vi "Set LEDs.vi"(8 "error in (no error)":errorcluster, 10 "LED Array":u32[][](array[colorbox]), 11 "LINX-SenseHat in":refnum<class "LINX-SenseHat.lvclass">) -> (0 "error out":errorcluster, 3 "LINX-SenseHat out":refnum<class "LINX-SenseHat.lvclass">)   [LabVIEW 2020, in "LINX-SenseHat.lvclass"]
uses:
  LINX-SenseHat.lvclass
  LINX-SenseHat.lvclass/LINX-SenseHat.ctl
  LINX I2C/LINX I2C.lvclass
panel:
  out "size(s)":i32
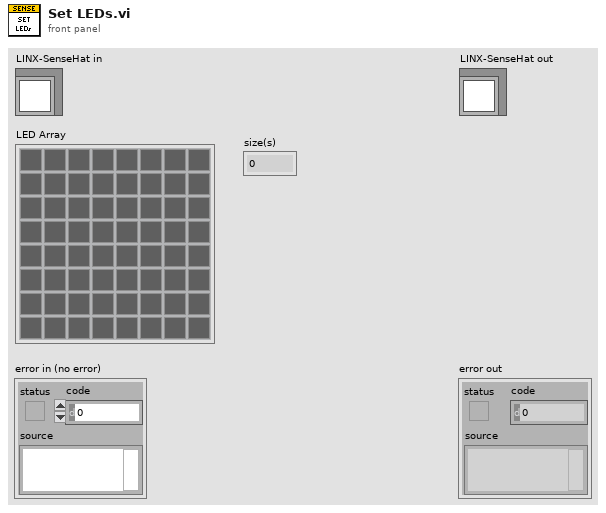
[diagram p1: front panel]
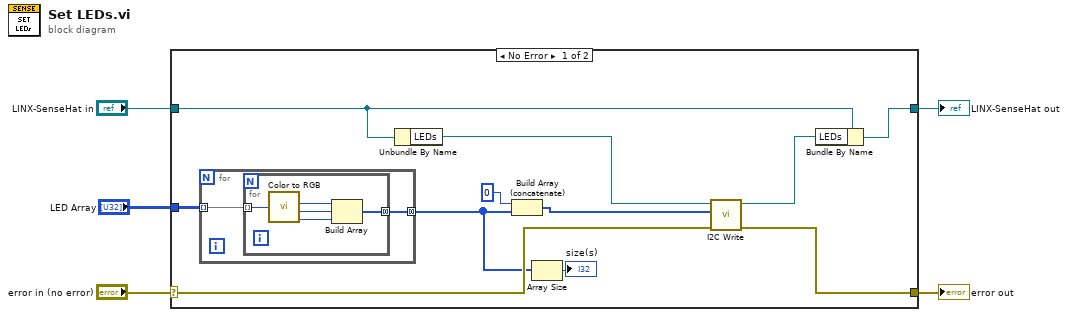
[diagram p0: block diagram]
diagram:
  n1 = case shown="No Error" "error in (no error)" {
    selector: "error in (no error)" -> [w12 w25]
    tunnel: [w11 w25] -> w4
    tunnel: [w13 w24] -> w2
    tunnel: "LINX-SenseHat in" -> [w14 w24]
    tunnel: "LED Array" -> [w7 _]
    frame No Error {
      n2 = for {
        tunnel: w7 -> [w18] mode=indexing
        tunnel: [w17] -> w9 mode=concatenating
        n3 = for {
          tunnel: w18 -> [w23] mode=indexing
          tunnel: [w19] -> w17 mode=concatenating
          n4 = call <vilib>:"Color to RGB.vi"("Color"=w23) -> ("R"=w22:u8, "G"=w21:u8, "B"=w20:u8)  [unwired: 1 out]
          n5 = Build Array(w22, w21, w20) -> (w19:u8[])
        }
      }
      n6 = Unbundle By Name(w14) -> ("LEDs"=w16:refnum<class "LINX I2C.lvclass">)
      n7 = Build Array (concatenate)(u8 0, w9) -> (w10:u8[])
      n8 = Array Size(array=w9) -> (size(s)=→"size(s)":i32)
      n9 = call "I2C Write.vi"("error in (no error)"=w12, "Bytes to Write"=w10, "LINX I2C in"=w16) -> ("error out"=w11:errorcluster, "LINX I2C out"=w15:refnum<class "LINX I2C.lvclass">)  [unwired: 7 in]
      n10 = Bundle By Name(cluster=w14, "LEDs"=w15) -> (w13:refnum<class "LINX-SenseHat.lvclass">)
    }
    frame Error {
    }
  }
  "error out" <- w4
  "LINX-SenseHat out" <- w2
